vi "Get Wait Until Data.vi"(8 "error in (no error)":errorcluster, 9 "Message":string="Send to Sequence", 10 "Sequence Data Queue":refnum<queue>, 11 "Queue in":refnum<queue>) -> (0 "error out":errorcluster, 2 "Data":dbl)   [LabVIEW 2018, in "Sequencing Library.lvlib"]
uses:
  Sequencing Library.lvlib
  support/Message Queue/Message Cluster.ctl
  support/Message Queue/Enqueue Message (Single).vi
  support/Message Queue/Message Queue.lvlib
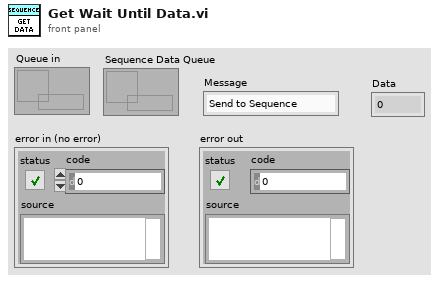
[diagram p1: front panel]
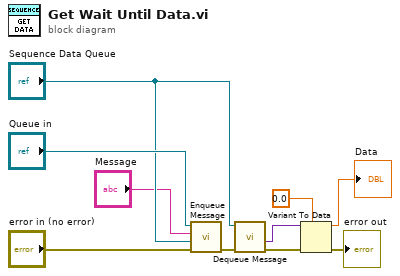
[diagram p0: block diagram]
diagram:
  n1 = call-poly "Enqueue Message.vi"("error in (no error)"="error in (no error)", "Message Data"="Sequence Data Queue", "Message"="Message", "Message Queue"="Queue in") -> ("error out"=w3:errorcluster)  [unwired: 6 in, 1 out]
  n2 = call "Dequeue Message.vi"("error in (no error)"=w3, "Message Queue"="Sequence Data Queue") -> ("error out"=w5:errorcluster, "Message Data"=w8:variant)  [unwired: 6 in, 2 out]
  n3 = Variant To Data(error in=w5, type=0.0, Variant=w8) -> (data=→"Data":dbl, error out=→"error out":errorcluster)
